vi "Set FPGA and generate single photons.vi"(8 "error in (no error)":errorcluster, 10 "Entrainment":bool, 11 "Photon #":i32) -> (0 "error out":errorcluster)   [LabVIEW 2013]
uses:
  <vilib>/DAQmx/write.llb/DAQmx Write (Digital Bool 1Line 1Point).vi
  <vilib>/DAQmx/read.llb/DAQmx Read (Digital Bool 1Line 1Point).vi
  <vilib>/DAQmx/miscellaneous.llb/DAQmx Fill In Error Info.vi
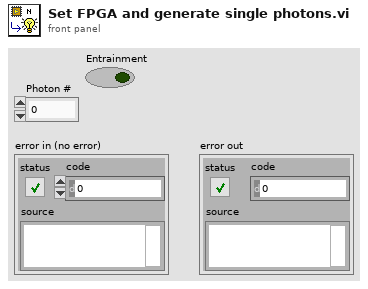
[diagram p1: front panel]
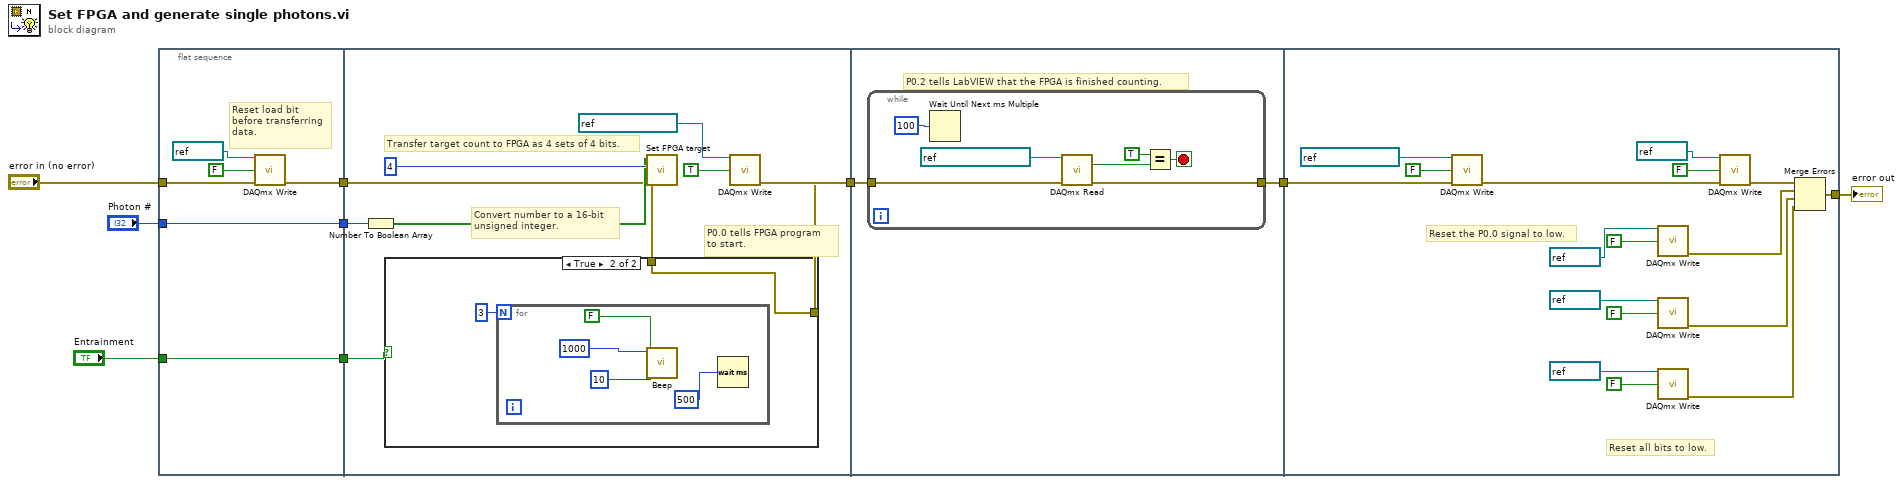
[diagram p0: block diagram]
diagram:
  n1 = flat-sequence {
    tunnel: "error in (no error)" -> [w12]
    tunnel: "Photon #" -> [w15]
    tunnel: [w15] -> w9
    tunnel: [w11] -> w8
    tunnel: [w10] -> w2
    tunnel: "Entrainment" -> [w10]
    tunnel: [w19] -> w7
    tunnel: w9 -> [w25]
    tunnel: w8 -> [w22]
    tunnel: w2 -> [w18]
    tunnel: w7 -> [w34]
    tunnel: [w33] -> w6
    tunnel: [w42] -> w4
    tunnel: w6 -> [w48]
    frame #0 {
      # "Reset load bit\nbefore transferring\ndata."
      n2 = call-poly <vilib>:"DAQmx Write.vi"("task/channels in"=refnum<k21> "BIT5", "data"=FALSE, "error in"=w12) -> ("error out"=w11:errorcluster)  [unwired: 10 in, 2 out]
    }
    frame #1 {
      # "P0.0 tells FPGA program \nto start."
      # "Convert number to a 16-bit\nunsigned integer."
      # "Transfer target count to FPGA as 4 sets of 4 bits."
      n3 = Number To Boolean Array(number=w25) -> (Boolean array=w23:bool[])
      n4 = call "Set FPGA target.vi"("error in (no error)"=w22, "Number of bits"=4, "Boolean array"=w23) -> ("error out"=w17:errorcluster)  [unwired: 8 in]
      n5 = case shown="True" w18 {
        tunnel: w17 -> [w26 w27]
        tunnel: [w26 w27] -> w16
        frame False {
        }
        frame True {
          n6 = for {
            N: 3 -> [_]
            n7 = call <vilib>:"Beep.vi"("use system alert? (T)"=FALSE, "duration (msec)"=u32 10, "frequency (Hz)"=u32 1000) -> ()  [unwired: 9 in]
            n8 = Wait (ms)(milliseconds to wait=u32 500) -> ()  [unwired: 1 out]
          }
        }
      }
      n9 = call-poly <vilib>:"DAQmx Write.vi"("task/channels in"=refnum<k21> "LaserChannel", "data"=TRUE, "error in"=w16) -> ("error out"=w19:errorcluster)  [unwired: 10 in, 2 out]
    }
    frame #2 {
      # "P0.2 tells LabVIEW that the FPGA is finished counting."
      n10 = while {
        tunnel: w34 -> [w40]
        tunnel: [w39] -> w33
        stop <- w36 stop-if-true
        n11 = Wait Until Next ms Multiple(millisecond multiple=u32 100) -> ()  [unwired: 1 out]
        n12 = call-poly <vilib>:"DAQmx Read.vi"("task/channels in"=refnum<k21> "P02countSignal", "error in"=w40) -> ("data"=w37:bool, "error out"=w39:errorcluster)  [unwired: 11 in, 1 out]
        n13 = Equal?(x=TRUE, y=w37) -> (x = y?=w36:bool)
      }
    }
    frame #3 {
      # "Reset all bits to low."
      # "Reset the P0.0 signal to low."
      n14 = call-poly <vilib>:"DAQmx Write.vi"("task/channels in"=refnum<k21> "LaserChannel", "data"=FALSE, "error in"=w48) -> ("error out"=w47:errorcluster)  [unwired: 10 in, 2 out]
      n15 = call-poly <vilib>:"DAQmx Write.vi"("task/channels in"=refnum<k21> "BIT2", "data"=FALSE) -> ("error out"=w55:errorcluster)  [unwired: 11 in, 2 out]
      n16 = call-poly <vilib>:"DAQmx Write.vi"("task/channels in"=refnum<k21> "BIT3", "data"=FALSE) -> ("error out"=w54:errorcluster)  [unwired: 11 in, 2 out]
      n17 = call-poly <vilib>:"DAQmx Write.vi"("task/channels in"=refnum<k21> "BIT4", "data"=FALSE) -> ("error out"=w53:errorcluster)  [unwired: 11 in, 2 out]
      n18 = call-poly <vilib>:"DAQmx Write.vi"("task/channels in"=refnum<k21> "BIT1", "data"=FALSE, "error in"=w47) -> ("error out"=w56:errorcluster)  [unwired: 10 in, 2 out]
      n19 = Merge Errors(w56, w55, w54, w53) -> (w42:errorcluster)
    }
  }
  "error out" <- w4
